vi "Return client handle.vi"(8 "error in (no error)":errorcluster, 9 "headers":T1[](array[typedef]), 10 "Client Handle":refnum<class "Abstract HTTP Client.lvclass">, 11 "REST Client in":refnum<class "REST Client.lvclass">) -> (0 "error out":errorcluster, 3 "REST Client out":refnum<class "REST Client.lvclass">)   [LabVIEW 2020, in "REST Client.lvlib" / "REST Client.lvclass"]
uses:
  REST Client.lvclass
  REST Client.lvclass/REST Client.ctl
  HTTP Header.ctl
  <vilib>/NI/Advanced HTTP Client/Header--Combo Box.ctl
  <vilib>/NI/Advanced HTTP Client/Session.lvclass
  <vilib>/VIPM Community/HTTP Client Plugin - Base/Classes/Abstract HTTP Client/Abstract HTTP Client.lvclass
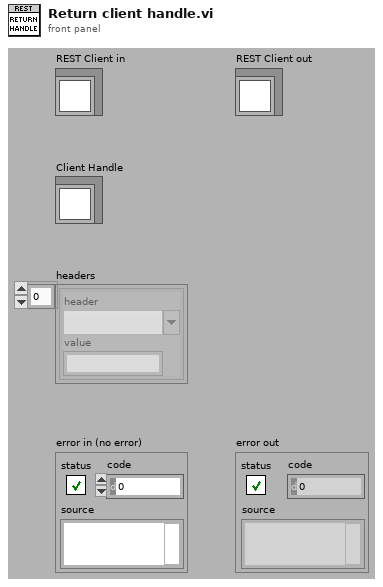
[diagram p1: front panel]
types:
  T1 = typedef "REST Client.lvlib/REST Client.lvclass/HTTP Header.ctl" = cluster{"header":T2, "value":string}
  T2 = typedef "lib_NI_Advanced HTTP Client.lvlib/Session.lvclass/Header--Combo Box.ctl" = string
  T3 = cluster{"Client Handle":refnum<class "Abstract HTTP Client.lvclass">, "headers":T1[]}
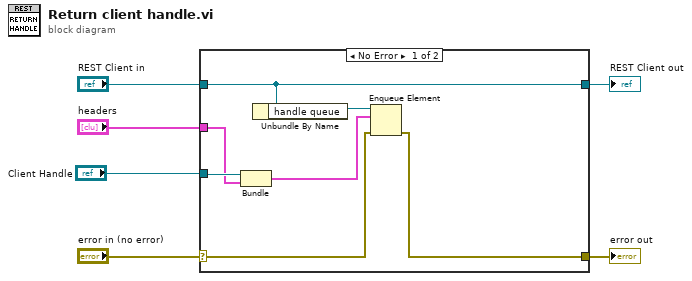
[diagram p0: block diagram]
diagram:
  n1 = case shown="No Error" "error in (no error)" {
    selector: "error in (no error)" -> [w9 w14]
    tunnel: [w8 w14] -> w5
    tunnel: [w11 w15] -> w3
    tunnel: "REST Client in" -> [w11 w15]
    tunnel: "Client Handle" -> [w13 _]
    tunnel: "headers" -> [w12 _]
    frame No Error {
      n2 = Bundle("Client Handle"=w13, "headers"=w12) -> (w7:T3)  [unwired: 1 in]
      n3 = Unbundle By Name(w11) -> ("handle queue"=w10:refnum<queue>)
      n4 = Enqueue Element(queue=w10, element=w7, error in (no error)=w9) -> (error out=w8:errorcluster)  [unwired: 1 in, 2 out]
    }
    frame Error {
    }
  }
  "error out" <- w5
  "REST Client out" <- w3
